vi "Save bline to memory2.vi"(0 "PSOCTSpectral Bline":u16[](array[numeric]), 1 "action":T1=enum."Save(ThorOCT)", 5 "index (row)":i32, 9 "PSOCT Spatial Bline":sgl[](array[numeric]), 11 "error in":errorcluster) -> (15 "error out":errorcluster)   [LabVIEW 2018]
uses:
  Controls/Save Bline to Mem Control.ctl
  Controls/FGV Actions.ctl
  Controls/Queue Manager Actions.ctl
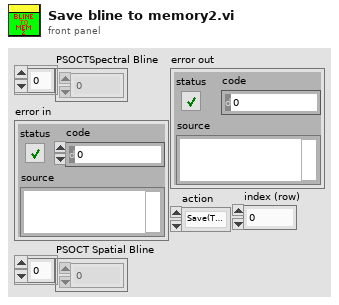
[diagram p1: front panel]
types:
  T1 = typedef "Save Bline to Mem Control.ctl" = enum16{"Output data", "Save(ThorOCT)", "Save(PSOCT)", "FFT and Save", "Uninit", "PSOCT Spectral buffer Set", "PSOCT Spatial buffer Set", "PSOCT Spectral buffer Init", "PSOCT Spatial buffer Init", "ThorOCT Spectral buffer Init", "ThorOCT Spatial buffer Init", "ThorOCT Spectral buffer Set", "ThorOCT Spatial buffer Set", "ThorOCT Spectral Save", "Alazar Spectral Save", "PSOCT save all", "Average"}
  T2 = typedef "FGV Actions.ctl" = enum16{"Init", "Set", "Get", "Clear"}
  T3 = typedef "System Parameters.ctl" = cluster{"Optical Parameters":T4, "Vibratome":T5, "Table Stages":T7, "Imaging Parameter":T10, "Galvo HW Parameters":cluster{"Analog Out Channel":tag, "Min Voltage":dbl, "Max Voltage":dbl, "Pixel Clock Source":tag, "Sample Rate":dbl, "Line Clock Out Ch":tag, "2P ready check":tag}, "Alazar parameters":T12, "Mosaic Paramter":cluster{"X Axis":cluster{"Start [mm]":dbl, "Steps [pts]":dbl, "End [mm]":dbl}, "Y Axis":cluster{"Start [mm]":dbl, "Steps [pts]":dbl, "End [mm]":dbl}, "Scan Pattern":enum16{"Uni-directional", "Bi-Directional", "Spiral Out", "Spiral In"}, "Overlap Options":cluster{"Overlap Type":enum16{"No Overlap", "X Only", "Y Only", "X and Y"}, "Percent Overlap":u8, "Justify":enum16{"Start", "Center", "End"}}}, "Manual Controls":T19, "Z stage setting":T23, "Attenuator":T24}
  T4 = typedef "Optical Parameters.ctl" = cluster{"Obj. Focal Length [mm]":dbl, "Scan Lens EFL[mm]":dbl, "Tube Lens EFL[mm]":dbl, "Galvo V Range (+/-)":dbl, "Galvo Max Half Angle [Deg]":dbl, "Max Galvo Range[%]":dbl}
  T5 = typedef "Vibratome Parameters.ctl" = cluster{"Pre Cut Dwell [s]":dbl, "Blade Frequency [RPM]":u16, "Slice Speed [mm/s]":dbl, "Post Cut Dwell [s]":dbl, "Ramp Time [s]":dbl, "Start X [mm]":dbl, "Start Y [mm]":dbl, "Slice Length [mm]":dbl, "Slice Axis":enum16{"X Axis", "Y Axis", "Z Axis"}, "Controller VISA Ref":refnum<visa-resource-name>, "Blade Frequency [Hz]":u16, "Analog Out Channel":tag, "Pixel Clock Source":tag, "Vib version":T6}
  T6 = typedef "vibratome.ctl" = enum16{"Vibratome1", "Vibratome3"}
  T7 = typedef "Translation Stage Parameters.ctl" = cluster{"X Stage":T8, "Y Stage":T8, "Z Stage":T8, "Attenuator":T8}
  T8 = typedef "Translation Stage Cluster.ctl" = cluster{"Position":dbl, "Is.Enabled?":bool, "Is.Connected?":bool, "Device SN":string, "AccelerationMaximum":dbl, "VelocityMaximum":dbl, "Acceleration":dbl, "Velocity":dbl, "waitTimeout (ms)":i32, "Model":T9, "Is.Homed?":bool, "MOVE":bool}
  T9 = typedef "Translation Stage Types.ctl" = enum16{"None", "Thorlabs LTS", "Thorlabs MLJ"}
  T10 = typedef "Imaging Parameters.ctl" = cluster{"Raster Scan Direction":T11, "Pixel Dwell Time [Clock Cycles]":u16, "Flyback Time [Clock Cycles]":u16, "XY Center [um]":cluster{"X":dbl, "Y":dbl}, "Pixel Step Size [um] X":dbl, "XY Image Size":enum16{"32 x 32", "64 x 64", "128 x 128", "256 x 256", "512 x 512", "1024 x 1024", "2048 x 2048"}, "Custom":bool, "Custom Size":cluster{"X":u16, "Y":u16}, "Line Averages":u16, "Pixel Step Size [um] Y":dbl}
  T11 = typedef "Scan Direction.ctl" = enum16{"Uni Directional", "Bi Directional", "None"}
  T12 = typedef "Alazar parameters.ctl" = cluster{"Trigger Settings":cluster{"General Trigger Settings":T13, "Trigger Engine 1":T14, "Trigger Engine 2":T14}, "Device ID":T15, "Ch A Input Control":T16, "Ch B Input Control":T16, "Acq Settings":T17, "Capture Clock":T18}
  T13 = typedef "General Trigger Settings.ctl" = cluster{"Trigger Operation":u32, "Coupling ID":u32, "Range ID":u32, "Delay":u32, "Timeout Ticks":u32, "Mode":u32, "Parameter":u32}
  T14 = typedef "Trigger Engine Controls.ctl" = cluster{"Trigger Engine":u32, "Source":u32, "Slope":u32, "Level":u32}
  T15 = typedef "Alazar Device ID.ctl" = cluster{"System ID":u32, "Board ID":u32}
  T16 = typedef "Channel Input Controls.ctl" = cluster{"Channel":u8, "Coupling":u32, "Range":u32, "Impedance":u32}
  T17 = typedef "Alazar Acquisition Settings.ctl" = cluster{"Record Length":u32, "Offset":u32, "Records Per Buffer":u32, "Records Count (Records/Acq)":u32, "Window Type":u32, "Footer":u32, "Samples per record":u32, "Output Format":u32}
  T18 = typedef "Clock Controls.ctl" = cluster{"Sample Rate":u32, "Decimation":u32, "Source":u32, "Edge":u32}
  T19 = typedef "Manual Controls.ctl" = cluster{"Data Path":path, "Save parameters":T20, "Acquisition mode":T21, "PSOCT Channel":u32, "Save data?":bool, "AIP rotation angle":dbl, "Pause acquisition?":bool, "Outgoing Mail Server (SMTP)":string, "Email":string, "Password":string, "Carrier 1":enum16{"T-Mobile", "AT&T", "Verizon", "Sprint"}, "phone number 1":string, "Subject":string, "Message":string, "Carrier 2":enum16{"T-Mobile", "AT&T", "Verizon", "Sprint"}, "phone number 2":string, "Check boundary?":bool, "Threshold":sgl, "Outputs for GPU FFT":T22, "Slice# init":i32}
  T20 = typedef "FFT parameters.ctl" = cluster{"start pixel":i32, "#pixels to save":i32}
  T21 = typedef "FFT mode.ctl" = enum16{"ThorOCT B line", "ThorOCT Spectral", "ThorOCT FFT", "Alazar B line", "Alazar FFT", "GPU FFT", "Alazar Spectral", "Simulation", "auto adjust focus", "Save all"}
  T22 = typedef "GPU FFT outputs.ctl" = enum16{"Amp + Phase diff", "Amp + Phase", "Amp only"}
  T23 = typedef "Vibratome Param.ctl" = cluster{"first cut height(mm)":dbl, "slice thickness[um]":dbl[], "#repetitions":u16, "image thickness(um)":dbl[], "#cycles per repetition":u16, "First image height(mm)":dbl, "Block?":bool[], "Z0":dbl, "fixed Z0?":bool}
  T24 = typedef "attenuator.ctl" = cluster{"Power after Objective (recalibrate every 6 month)":dbl[]}
  T25 = typedef "Queue Manager Actions.ctl" = enum16{"Init", "Enqueue", "Enqueue All", "Preview Queue", "Dequeue", "Get Status", "Flush Queue", "Flush All Queues", "Release All Queues", "Release Queue", "Enqueue at Opposite End"}
  T26 = typedef "Go Scan Actions.ctl" = enum16{"Init(ThorOCT Spatial)", "Init(ThorOCT Spectral)", "Init(GPU FFT)", "Init(Alazar FFT)", "Init Scan Head(ThorOCT Spectral)", "Init Scan Head(ThorOCT Spatial)", "Init Scan Head", "Init Table Stage", "Init Vibratome", "Generate Mosaic", "Generate Z Position", "Go to Image Z", "Go Image Home", "Go Mosaic", "Acquire Image(ThorOCT Spatial)", "Acquire Image(ThorOCT Spectral)", "Acquire Image(GPU FFT)", "Acquire Image(Alazar FFT)", "Go Vibratome", "Slice", "Finished(ThorOCT)", "Finished", "Init(Alazar Spectral)", "Go Vibratome3", "Tissue boundary"}
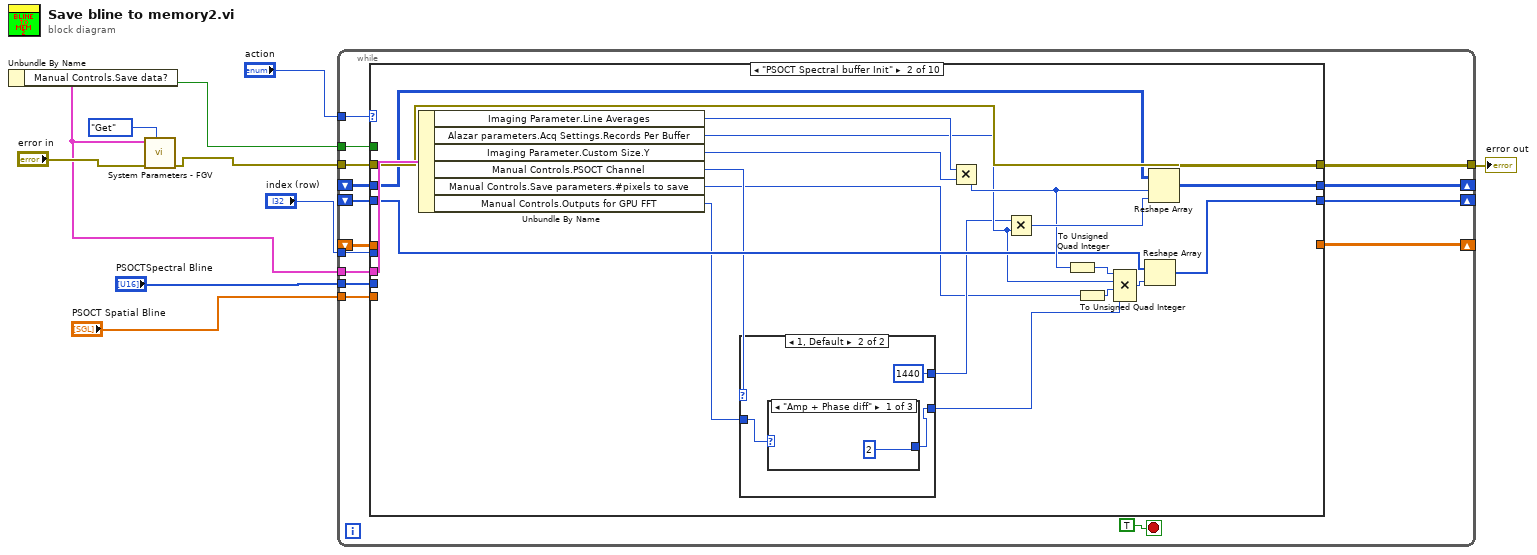
[diagram p0: block diagram]
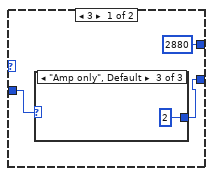
[diagram p3: hidden frame]
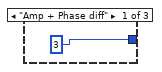
[diagram p4: hidden frame]
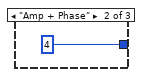
[diagram p5: hidden frame]
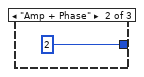
[diagram p6: hidden frame]
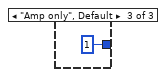
[diagram p7: hidden frame]
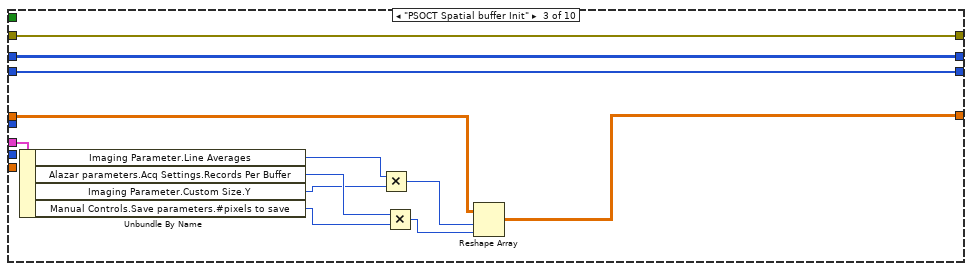
[diagram p8: hidden frame]
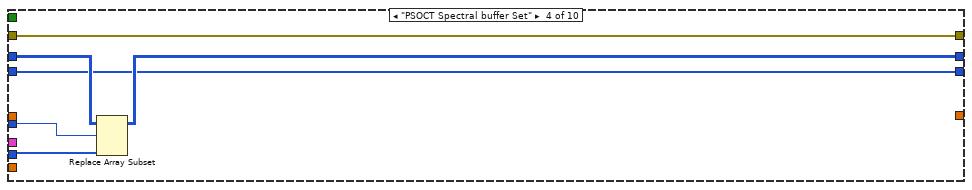
[diagram p9: hidden frame]
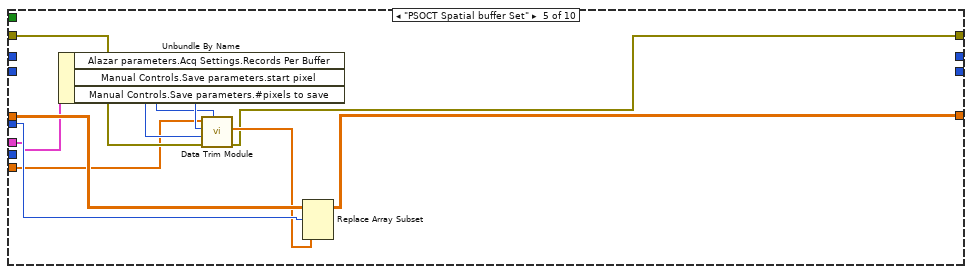
[diagram p10: hidden frame]
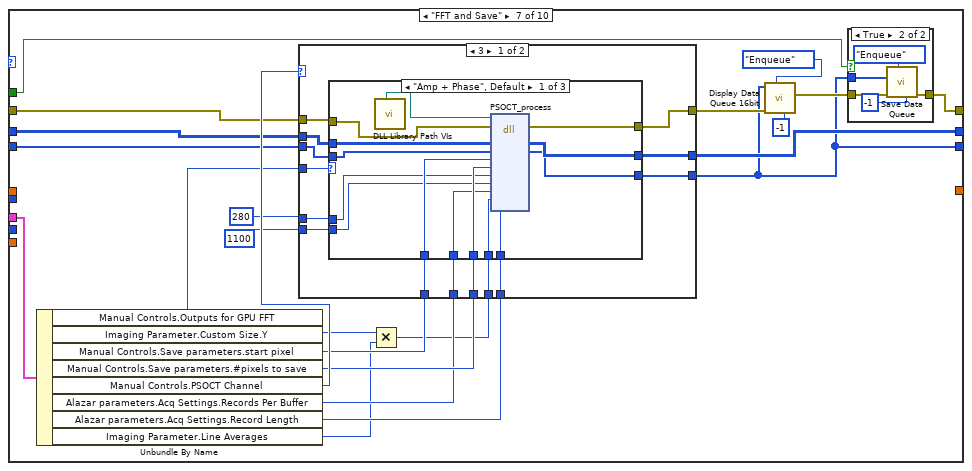
[diagram p12: hidden frame]
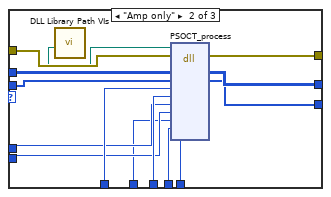
[diagram p13: hidden frame]
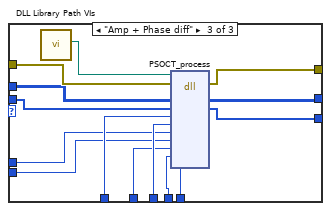
[diagram p14: hidden frame]
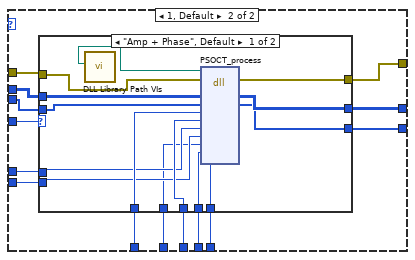
[diagram p15: hidden frame]
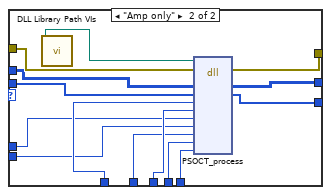
[diagram p16: hidden frame]
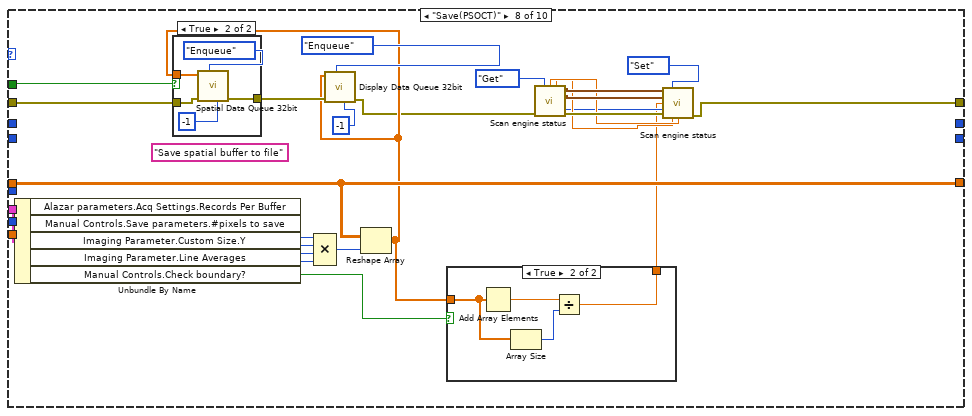
[diagram p18: hidden frame]
diagram:
  n1 = call "System Parameters - FGV.vi"("Actions"=FGV_Actions."Get", "Error In"="error in") -> ("Error Out"=w3:errorcluster, "System Parameters [Out]"=w2:T3)  [unwired: 8 in]
  n2 = Unbundle By Name(w2) -> ("Manual Controls.Save data?"=w1:bool)
  n3 = while {
    tunnel: "action" -> [w25]
    shift-right: [w24] -> _
    shift-left: _ -> [w23]
    tunnel: "PSOCTSpectral Bline" -> [w22]
    tunnel: "index (row)" -> [w20]
    tunnel: w3 -> [w19]
    tunnel: w2 -> [w18]
    tunnel: [w17] -> w6
    shift-right: [w16] -> _
    shift-left: _ -> [w15]
    tunnel: "PSOCT Spatial Bline" -> [w14]
    tunnel: w1 -> [w13]
    shift-right: [w12] -> _
    shift-left: _ -> [w11]
    stop <- TRUE stop-if-true
    n4 = case shown="\"PSOCT Spectral buffer Init\"" w25 {
      tunnel: [w29 w47 w63 w75 _ _ w99 _ _ w277] -> w24
      tunnel: w23 -> [w29 w38 w63 w78 _ _ w108 _ _ w277]
      tunnel: w22 -> [_ _ _ w76 _ _ _ _ _ _]
      tunnel: w20 -> [_ _ _ w77 w87 _ _ _ _ _]
      tunnel: w19 -> [w27 w43 w64 w74 w83 w90 w109 w241 w259 w280]
      tunnel: w18 -> [_ w46 w71 _ w84 _ w112 w239 w274 _]
      tunnel: [w27 w43 w64 w74 w79 w90 w98 w218 w252 w279] -> w17
      tunnel: [w28 _ w68 _ w88 _ _ w240 w275 _] -> w16
      tunnel: w15 -> [w28 _ w61 _ w89 _ _ w240 w275 _]
      tunnel: w14 -> [_ _ _ _ w81 _ _ _ _ _]
      tunnel: w13 -> [_ _ _ _ _ _ w111 w231 _ _]
      tunnel: [w26 w42 w62 w73 _ _ w94 _ _ w276] -> w12
      tunnel: w11 -> [w26 w37 w62 w73 _ _ w107 _ _ w276]
      frame Default {
      }
      frame "PSOCT Spectral buffer Init" {
        n5 = Unbundle By Name(w46) -> ("Imaging Parameter.Line Averages"=w45:u16, "Alazar parameters.Acq Settings.Records Per Buffer"=w35:u32, "Imaging Parameter.Custom Size.Y"=w44:u16, "Manual Controls.PSOCT Channel"=w32:u32, "Manual Controls.Save parameters.#pixels to save"=w31:i32, "Manual Controls.Outputs for GPU FFT"=w30:T22)
        n6 = case shown="1, Default" w32 {
          tunnel: [w51 w57] -> w39
          tunnel: w30 -> [w50 w56]
          tunnel: [u32 2880 ("element") u32 1440 ("element")] -> w33
          frame 3 {
            n7 = case shown="\"Amp only\", Default" w50 {
              tunnel: [3 u64 4 ("element") u64 2 ("element")] -> w51
              frame "Amp + Phase diff" {
              }
              frame "Amp + Phase" {
              }
              frame "Amp only", Default {
              }
            }
          }
          frame 1, Default {
            n8 = case shown="\"Amp + Phase diff\"" w56 {
              tunnel: [2 u64 2 ("element") u64 1 ("element")] -> w57
              frame "Amp + Phase diff" {
              }
              frame "Amp + Phase" {
              }
              frame "Amp only", Default {
              }
            }
          }
        }
        n9 = Multiply(x=w45, y=w44) -> (x*y=w41:u16)
        n10 = Multiply(x=w33, y=w35) -> (x*y=w48:u32)
        n11 = To Unsigned Quad Integer(1:w41) -> (0:w36:u64)
        n12 = To Unsigned Quad Integer(1:w31) -> (0:w34:u64)
        n13 = Compound Arithmetic op=MULTIPLY(w36, w35, w34, w39) -> (w40:u64)
        n14 = Reshape Array(w37, w40) -> (w42:u16[])
        n15 = Reshape Array(w38, w41, w48) -> (w47:u16[][])
      }
      frame "PSOCT Spatial buffer Init" {
        n16 = Unbundle By Name(w71) -> ("Imaging Parameter.Line Averages"=w67:u16, "Alazar parameters.Acq Settings.Records Per Buffer"=w69:u32, "Imaging Parameter.Custom Size.Y"=w66:u16, "Manual Controls.Save parameters.#pixels to save"=w70:i32)
        n17 = Multiply(x=w67, y=w66) -> (x*y=w65:u16)
        n18 = Multiply(x=w69, y=w70) -> (x*y=w72:u32)
        n19 = Reshape Array(w61, w65, w72) -> (w68:sgl[][])
      }
      frame "PSOCT Spectral buffer Set" {
        n20 = Replace Array Subset(array=w78, new element=w76, index (row)=w77) -> (w75:u16[][])  [unwired: 1 in]
      }
      frame "PSOCT Spatial buffer Set" {
        n21 = Unbundle By Name(w84) -> ("Alazar parameters.Acq Settings.Records Per Buffer"=w86:u32, "Manual Controls.Save parameters.start pixel"=w85:i32, "Manual Controls.Save parameters.#pixels to save"=w80:i32)
        n22 = call "Data Trim Module.vi"("#pixels to save"=w80, "error in"=w83, "start pixel"=w85, "#A-lines"=w86, "1D Array in"=w81) -> ("error out"=w79:errorcluster, "array for saving"=w82:sgl[])  [unwired: 5 in]
        n23 = Replace Array Subset(array=w89, new element=w82, index (row)=w87) -> (w88:sgl[][])  [unwired: 1 in]
      }
      frame "Uninit" {
      }
      frame "FFT and Save" {
        n24 = Unbundle By Name(w112) -> ("Manual Controls.Outputs for GPU FFT"=w100:T22, "Imaging Parameter.Custom Size.Y"=w93:u16, "Manual Controls.Save parameters.start pixel"=w106:i32, "Manual Controls.Save parameters.#pixels to save"=w105:i32, "Manual Controls.PSOCT Channel"=w110:u32, "Alazar parameters.Acq Settings.Records Per Buffer"=w102:u32, "Alazar parameters.Acq Settings.Record Length"=w101:u32, "Imaging Parameter.Line Averages"=w92:u16)
        n25 = Multiply(x=w93, y=w92) -> (x*y=w91:u16)
        n26 = case shown="3" w110 {
          tunnel: w109 -> [w126 w182]
          tunnel: w108 -> [w125 w181]
          tunnel: w107 -> [w124 w180]
          tunnel: w106 -> [w123 w179]
          tunnel: w105 -> [w122 w178]
          tunnel: i16 280 ("a") -> [w121 w177]
          tunnel: i16 1100 ("b") -> [w120 w176]
          tunnel: w102 -> [w119 w175]
          tunnel: w91 -> [w118 w174]
          tunnel: w101 -> [w117 w173]
          tunnel: [w114 w170] -> w96
          tunnel: [w113 w169] -> w99
          tunnel: [w116 w172] -> w94
          tunnel: w100 -> [w115 w171]
          frame 3 {
            n27 = case shown="\"Amp + Phase\", Default" w115 {
              tunnel: w126 -> [w140 w154 w168]
              tunnel: w125 -> [w137 w151 w167]
              tunnel: w124 -> [w136 w150 w166]
              tunnel: w123 -> [w135 w149 w165]
              tunnel: w122 -> [w134 w148 w164]
              tunnel: w121 -> [w133 w147 w163]
              tunnel: w120 -> [w132 w146 w162]
              tunnel: w119 -> [w131 w145 w161]
              tunnel: w118 -> [w130 w144 w160]
              tunnel: w117 -> [w129 w143 w159]
              tunnel: [w128 w142 w158] -> w114
              tunnel: [w139 w153 w157] -> w113
              tunnel: [w138 w152 w156] -> w116
              frame "Amp + Phase", Default {
                n28 = call "DLL Library Path VIs.vi"() -> ("GPU FFT amp amp phase phase"=w127:path)  [unwired: 5 in, 6 out]
                n29 = dll-call lib="C:/Project/SerialSectionOCT/SerialSectOCT/Labview Software/DLL/CUDA_FFT_2_channel_amp_amp_phase_phase.dll" fn="PSOCT_process"(path in=w127, error in=w140, "h_signal"=w137, "h_processed_signal"=w136, "Z0"=w135, "DEPTH"=w134, "a"=w133, "b"=w132, "NALINES"=w131, "NBLINES"=w130, "SAMPLES"=w129) -> (error out=w128:errorcluster, "h_signal"=w139:u16[][], "h_processed_signal"=w138:u16[])  [unwired: 9 in, 1 out]
              }
              frame "Amp only" {
                n30 = call "DLL Library Path VIs.vi"() -> ("GPU FFT amp amp"=w141:path)  [unwired: 5 in, 6 out]
                n31 = dll-call lib="C:/Project/SerialSectionOCT/SerialSectOCT/Labview Software/DLL/CUDA_FFT_2_channel_amp_amp.dll" fn="PSOCT_process"(path in=w141, error in=w154, "h_signal"=w151, "h_processed_signal"=w150, "Z0"=w149, "DEPTH"=w148, "a"=w147, "b"=w146, "NALINES"=w145, "NBLINES"=w144, "SAMPLES"=w143) -> (error out=w142:errorcluster, "h_signal"=w153:u16[][], "h_processed_signal"=w152:u16[])  [unwired: 9 in, 1 out]
              }
              frame "Amp + Phase diff" {
                n32 = call "DLL Library Path VIs.vi"() -> ("GPU FFT amp amp phase diff"=w155:path)  [unwired: 5 in, 6 out]
                n33 = dll-call lib="C:/Project/SerialSectionOCT/SerialSectOCT/Labview Software/DLL/CUDA_FFT_2_channel_amp_amp_phasediff.dll" fn="PSOCT_process"(path in=w155, error in=w168, "h_signal"=w167, "h_processed_signal"=w166, "Z0"=w165, "DEPTH"=w164, "a"=w163, "b"=w162, "NALINES"=w161, "NBLINES"=w160, "SAMPLES"=w159) -> (error out=w158:errorcluster, "h_signal"=w157:u16[][], "h_processed_signal"=w156:u16[])  [unwired: 9 in, 1 out]
              }
            }
          }
          frame 1, Default {
            n34 = case shown="\"Amp + Phase\", Default" w171 {
              tunnel: w182 -> [w196 w210]
              tunnel: w181 -> [w193 w209]
              tunnel: w180 -> [w192 w208]
              tunnel: w179 -> [w191 w207]
              tunnel: w178 -> [w190 w206]
              tunnel: w177 -> [w189 w205]
              tunnel: w176 -> [w188 w204]
              tunnel: w175 -> [w187 w203]
              tunnel: w174 -> [w186 w202]
              tunnel: w173 -> [w185 w201]
              tunnel: [w184 w200] -> w170
              tunnel: [w195 w199] -> w169
              tunnel: [w194 w198] -> w172
              frame "Amp + Phase", Default {
                n35 = call "DLL Library Path VIs.vi"() -> ("GPU FFT single amp phase"=w183:path)  [unwired: 5 in, 6 out]
                n36 = dll-call lib="C:/Project/SerialSectionOCT/SerialSectOCT/Labview Software/DLL/CUDA_FFT_1_channel_amp_phase.dll" fn="PSOCT_process"(path in=w183, error in=w196, "h_signal"=w193, "h_processed_signal"=w192, "Z0"=w191, "DEPTH"=w190, "a"=w189, "b"=w188, "NALINES"=w187, "NBLINES"=w186, "SAMPLES"=w185) -> (error out=w184:errorcluster, "h_signal"=w195:u16[][], "h_processed_signal"=w194:u16[])  [unwired: 9 in, 1 out]
              }
              frame "Amp only" {
                n37 = call "DLL Library Path VIs.vi"() -> ("GPU FFT single amp"=w197:path)  [unwired: 5 in, 6 out]
                n38 = dll-call lib="C:/Project/SerialSectionOCT/SerialSectOCT/Labview Software/DLL/CUDA_FFT_1_channel_amp.dll" fn="PSOCT_process"(path in=w197, error in=w210, "h_signal"=w209, "h_processed_amps"=w208, "Z0"=w207, "DEPTH"=w206, "a"=w205, "b"=w204, "NALINES"=w203, "NBLINES"=w202, "SAMPLES"=w201) -> (error out=w200:errorcluster, "h_signal"=w199:u16[][], "h_processed_amps"=w198:u16[])  [unwired: 9 in, 1 out]
              }
            }
          }
        }
        n39 = call "Display Data Queue 16bit.vi"("timeout in ms (-1)"=-1, "Action"=Queue_Manager_Actions."Enqueue", "data in"=w94) -> ()  [unwired: 5 in, 4 out]
        n40 = case shown="True" w111 {
          tunnel: w96 -> [w211 w216]
          tunnel: [w211 w215] -> w98
          tunnel: w94 -> [_ w212]
          frame False {
          }
          frame True {
            n41 = call "Save Data Queue.vi"("timeout in ms (-1)"=-1, "Action"=Queue_Manager_Actions."Enqueue", "error in (no error)"=w216, "data in"=w212) -> ("error out"=w215:errorcluster)  [unwired: 4 in, 3 out]
          }
        }
      }
      frame "Save(PSOCT)" {
        (unwired) "Save spatial buffer to file"
        n42 = Unbundle By Name(w239) -> ("Alazar parameters.Acq Settings.Records Per Buffer"=w238:u32, "Manual Controls.Save parameters.#pixels to save"=w237:i32, "Imaging Parameter.Custom Size.Y"=w236:u16, "Imaging Parameter.Line Averages"=w230:u16, "Manual Controls.Check boundary?"=w229:bool)
        n43 = Compound Arithmetic op=MULTIPLY(w238, w237, w236, w230) -> (w235:u32)
        n44 = Reshape Array(w240, w235) -> (w228:sgl[])
        n45 = case shown="True" w231 {
          tunnel: w241 -> [w246 w251]
          tunnel: [w246 w250] -> w234
          tunnel: w228 -> [_ w247]
          frame False {
          }
          frame True {
            n46 = call "Spatial Data Queue 32bit.vi"("timeout in ms (-1)"=-1, "Action"=Queue_Manager_Actions."Enqueue", "error in (no error)"=w251, "data in"=w247) -> ("error out"=w250:errorcluster)  [unwired: 4 in, 3 out]
          }
        }
        n47 = call "Display Data Queue 32bit.vi"("timeout in ms (-1)"=-1, "Action"=Queue_Manager_Actions."Enqueue", "error in (no error)"=w234, "data in"=w228) -> ("error out"=w219:errorcluster)  [unwired: 4 in, 3 out]
        n48 = case shown="True" w229 {
          tunnel: w228 -> [_ w242]
          tunnel: [_ w243] -> w217
          frame False {
          }
          frame True {
            n49 = Add Array Elements(numeric array=w242) -> (sum=w245:sgl)
            n50 = Array Size(array=w242) -> (size(s)=w244:i32)
            n51 = Divide(x=w245, y=w244) -> (x/y=w243:sgl)
          }
        }
        n52 = call "Scan engine status.vi"("Actions"=FGV_Actions."Get", "Error In"=w219) -> ("slice plane out"=w222:dbl, "image plane out"=w221:dbl, "XY Graph out"=w224:cluster{"X":dbl, "Y":dbl}[], "Current Position out"=w225:cluster{"X":dbl, "Y":dbl}, "Current state out"=w220:T26, "Error Out"=w226:errorcluster)  [unwired: 7 in, 1 out]
        n53 = call "Scan engine status.vi"("XY Graph in"=w224, "Actions"=FGV_Actions."Set", "Current Position in"=w225, "average"=w217, "Current state in"=w220, "Error In"=w226, "image plane"=w221, "slice plane"=w222) -> ("Error Out"=w218:errorcluster)  [unwired: 1 in, 6 out]
      }
      frame "Average" {
        (unwired) "Calculate average pixel value"
        n54 = Unbundle By Name(w274) -> ("Alazar parameters.Acq Settings.Records Per Buffer"=w273:u32, "Manual Controls.Save parameters.#pixels to save"=w272:i32, "Imaging Parameter.Custom Size.Y"=w271:u16, "Imaging Parameter.Line Averages"=w269:u16)
        n55 = Compound Arithmetic op=MULTIPLY(w273, w272, w271, w269) -> (w270:u32)
        n56 = call "Scan engine status.vi"("Actions"=FGV_Actions."Get", "Error In"=w259) -> ("slice plane out"=w261:dbl, "image plane out"=w260:dbl, "XY Graph out"=w263:cluster{"X":dbl, "Y":dbl}[], "Current Position out"=w264:cluster{"X":dbl, "Y":dbl}, "Current state out"=w257:T26, "Error Out"=w265:errorcluster)  [unwired: 7 in, 1 out]
        n57 = Reshape Array(w275, w270) -> (w253:sgl[])
        n58 = Add Array Elements(numeric array=w253) -> (sum=w268:sgl)
        n59 = Array Size(array=w253) -> (size(s)=w267:i32)
        n60 = Divide(x=w268, y=w267) -> (x/y=w258:sgl)
        n61 = call "Scan engine status.vi"("XY Graph in"=w263, "Actions"=FGV_Actions."Set", "Current Position in"=w264, "average"=w258, "Current state in"=w257, "Error In"=w265, "image plane"=w260, "slice plane"=w261) -> ("Error Out"=w254:errorcluster)  [unwired: 1 in, 6 out]
        n62 = call "Display Data Queue 32bit.vi"("timeout in ms (-1)"=-1, "Action"=Queue_Manager_Actions."Enqueue", "error in (no error)"=w254, "data in"=w253) -> ("error out"=w252:errorcluster)  [unwired: 4 in, 3 out]
      }
      frame "Alazar Spectral Save" {
        n63 = call "Spectral Save Queue.vi"("timeout in ms (-1)"=-1, "Action"=Queue_Manager_Actions."Enqueue", "error in (no error)"=w280, "data in"=w277) -> ("error out"=w279:errorcluster)  [unwired: 4 in, 3 out]
      }
    }
  }
  "error out" <- w6
